vi "WriteCalInfoToInst.vi"(9 "Enable":string, 10 "SN":string, 11 "TestInfo_In":string) -> (3 "TestInfo_Out":string)   [LabVIEW 2018]
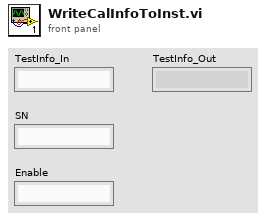
[diagram p1: front panel]
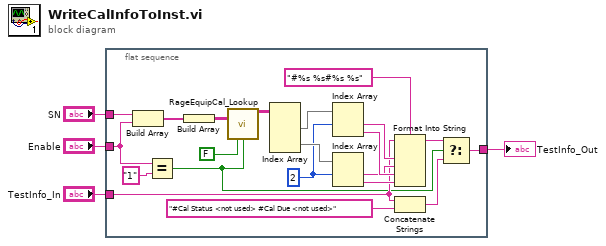
[diagram p0: block diagram]
diagram:
  n1 = flat-sequence {
    tunnel: "SN" -> [w14]
    tunnel: "Enable" -> [w13]
    tunnel: "TestInfo_In" -> [w10]
    tunnel: [w6] -> w4
    frame #0 {
      w16 = 2 ("index")
      n2 = Build Array(w14, w13) -> (w25:string[])
      n3 = Equal?(x=w13, y="1") -> (x = y?=w8:bool)
      n4 = Build Array(w25) -> (w24:string[][])
      n5 = call "RageEquipCal_Lookup.vi"("SN / Active(1=T)"=w24, "Use Popup Warning(T)"=FALSE ("Run Vi (T)"), "Run Vi (T)"=w8) -> ("Status Summary Out"=w23:string[][])  [unwired: 10 in, 2 out]
      n6 = Index Array(array=w23) -> (element #1=w22:string[], element #2=w21:string[])  [unwired: 4 in]
      n7 = Index Array(array=w22, index #1=w16) -> (element #1=w20:string, element #2=w19:string)  [unwired: 1 in]
      n8 = Index Array(array=w21, index #1=w16) -> (element #1=w17:string, element #2=w18:string)  [unwired: 1 in]
      n9 = Format Into String(format string="#%s %s#%s %s", initial string=w10, w20, w17, w19, w18) -> (resulting string=w9:string)  [unwired: 1 in, 1 out]
      n10 = Concatenate Strings(w10, "#Cal Status <not used> #Cal Due <not used>" ("format string")) -> (w7:string)
      n11 = Select(t=w9, s=w8, f=w7) -> (s? t:f=w6:string)
    }
  }
  "TestInfo_Out" <- w4
